vi "GVLT-FGV-Data.vi"(7 "State":T1, 8 "error in":errorcluster, 10 "Data In":dbl[][](array[numeric])) -> (0 "error out":errorcluster, 2 "Data Out":dbl[][](array[numeric]))   [LabVIEW 2023]
uses:
  Controls/GLVT-FGV-States.ctl
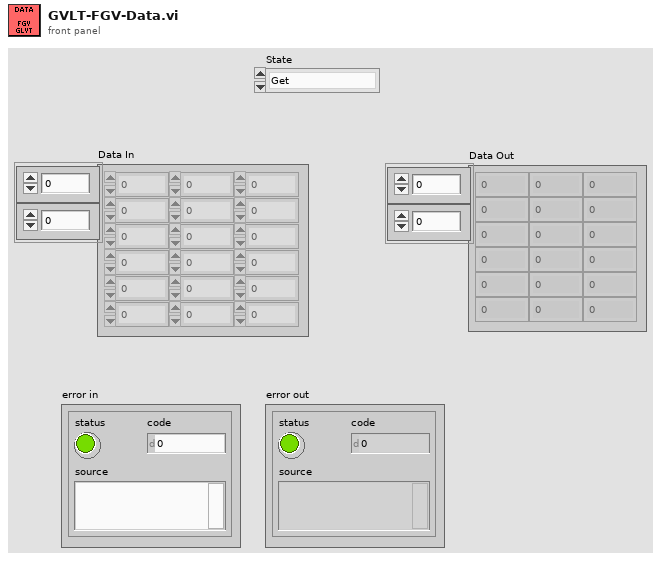
[diagram p1: front panel]
types:
  T1 = typedef "GLVT-FGV-States.ctl" = enum16{"Get", "Set"}
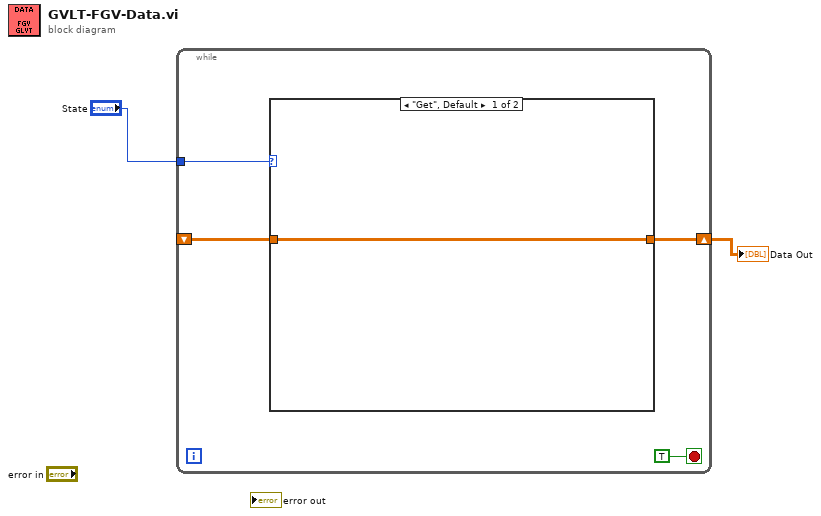
[diagram p0: block diagram]
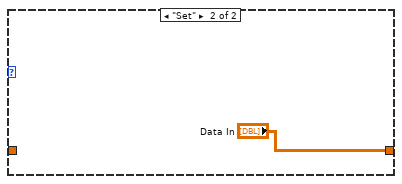
[diagram p2: hidden frame]
diagram:
  n1 = while {
    shift-right: [w4] -> w1
    shift-left: _ -> [w3]
    tunnel: "State" -> [w5]
    stop <- TRUE stop-if-true
    n2 = case shown="\"Get\", Default" w5 {
      tunnel: [w7 "Data In"] -> w4
      tunnel: w3 -> [w7 _]
      frame "Get", Default {
      }
      frame "Set" {
      }
    }
  }
  "Data Out" <- w1
